vi "convert from time clust to ns.vi"(7 "time cluster":T1={"day"=0, "hour"=0, "min"=0, "sec"=1, "msec"=0, "usec"=0, "nsec"=0}) -> (8 "time (nsec)":i64=1000)   [LabVIEW 2014]
doc: "This subvi converts a typedefined U32 time cluster in a format of: [weeks, days, hours (24), min, sec, msec, usec, and nsec] to nsec \n\nIt uses a I64 format for the time in nsec and thus is limited to 2^63-1 nsec before rolling over, meaning that it wont reset for years.\n\nPaul K Dixon\nP350\nCSUSB Physics"
uses:
  typedefs/time cluster typedef.ctl
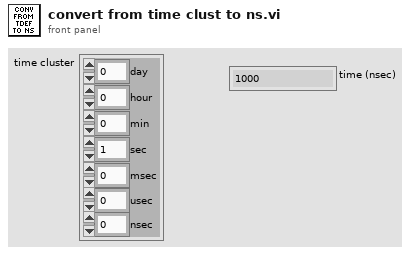
[diagram p1: front panel]
types:
  T1 = typedef "time cluster typedef.ctl" = cluster{"day":u32, "hour":u32, "min":u32, "sec":u32, "msec":u32, "usec":u32, "nsec":u32}
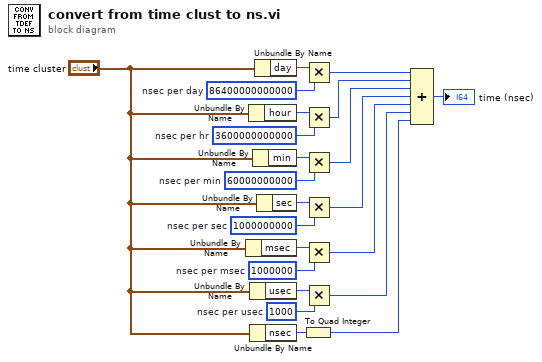
[diagram p0: block diagram]
diagram:
  w3 = i64 1000  # nsec per usec
  w8 = i64 1000000  # nsec per msec
  w15 = i64 1000000000  # nsec per sec
  w17 = i64 60000000000  # nsec per min
  w19 = i64 3600000000000  # nsec per hr
  w20 = i64 86400000000000  # nsec per day
  n1 = Unbundle By Name("time cluster") -> ("msec"=w9:u32)
  n2 = Unbundle By Name("time cluster") -> ("hour"=w22:u32)
  n3 = Unbundle By Name("time cluster") -> ("usec"=w4:u32)
  n4 = Unbundle By Name("time cluster") -> ("nsec"=w6:u32)
  n5 = Unbundle By Name("time cluster") -> ("min"=w18:u32)
  n6 = Unbundle By Name("time cluster") -> ("day"=w21:u32)
  n7 = Unbundle By Name("time cluster") -> ("sec"=w16:u32)
  n8 = To Quad Integer(1:w6) -> (0:w1:i64)
  n9 = Multiply(x=w21, y=w20) -> (x*y=w14:i64)
  n10 = Multiply(x=w22, y=w19) -> (x*y=w13:i64)
  n11 = Multiply(x=w18, y=w17) -> (x*y=w12:i64)
  n12 = Multiply(x=w16, y=w15) -> (x*y=w11:i64)
  n13 = Multiply(x=w9, y=w8) -> (x*y=w7:i64)
  n14 = Multiply(x=w4, y=w3) -> (x*y=w2:i64)
  n15 = Compound Arithmetic op=ADD(w14, w13, w12, w11, w7, w2, w1) -> (→"time (nsec)":i64)
